vi "Get Side Patterns.vi"(8 "error in (no error)":errorcluster, 11 "Tile in":refnum<class "Tile.lvclass">) -> (0 "error out":errorcluster, 2 "Sides":bool[][](array[boolean]), 3 "Tile out":refnum<class "Tile.lvclass">)   [LabVIEW 2020, in "Tile.lvclass"]
uses:
  Tile.lvclass
  Tile.lvclass/Tile.ctl
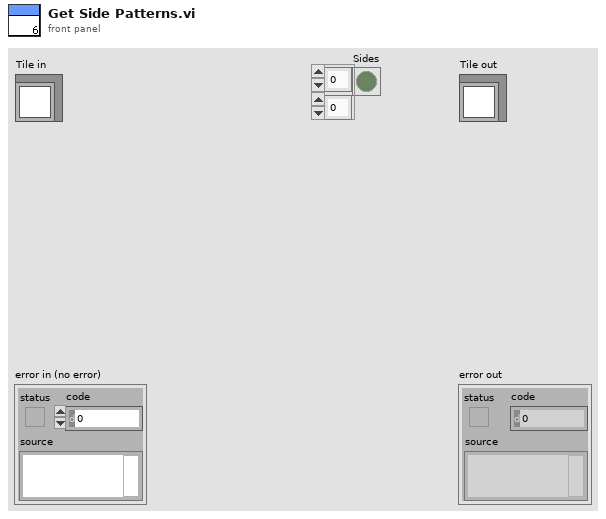
[diagram p1: front panel]
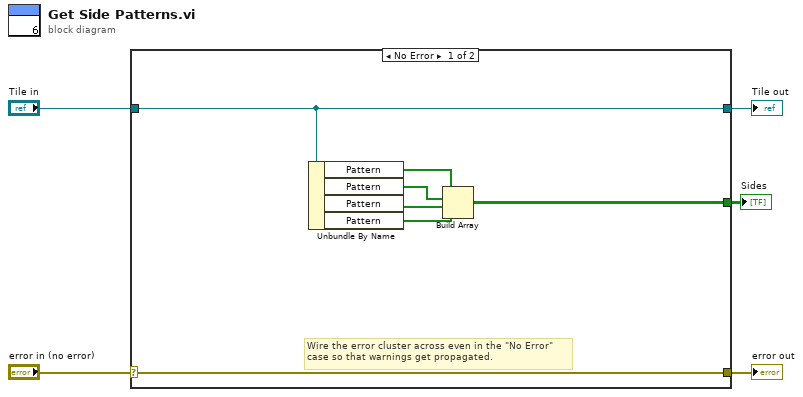
[diagram p0: block diagram]
diagram:
  n1 = case shown="No Error" "error in (no error)" {
    selector: "error in (no error)" -> [w12 w14]
    tunnel: [w12 w14] -> w4
    tunnel: [w11 w13] -> w2
    tunnel: "Tile in" -> [w11 w13]
    tunnel: [w6 _] -> w1
    frame No Error {
      # "Wire the error cluster across even in the \"No Error\"\ncase so that warnings get propagated."
      n2 = Unbundle By Name(w11) -> ("Pattern"=w7:bool[], "Pattern"=w8:bool[], "Pattern"=w9:bool[], "Pattern"=w10:bool[])
      n3 = Build Array(w7, w8, w9, w10) -> (w6:bool[][])
    }
    frame Error {
    }
  }
  "error out" <- w4
  "Tile out" <- w2
  "Sides" <- w1
